vi "DimIndicators.VI-Tree.vi"   [LabVIEW 2014, in "DimIndicators.lvlib"]
doc: "DimIndicators provides some easy to use indicators and controls for GUIs.\n\nHistory: 21-FEB-2006, Dietrich Beck\n\nCopyright (C)\nGesellschaft für Schwerionenforschung, GSI\nPlanckstr. 1\n64291 Darmstadt\nGermany\n\nContact: D.Beck@gsi.de \n\nThis program is free software; you can redistribute it and/or modify it under the terms of the GNU General Public License as published by the Free Software Foundation; either version 2 of the license, or (at your option) any later version.\n\nThis program is distributed in the hope that it will be useful, but WITHOUT ANY WARRANTY; without even the implied warranty of MERCHANTABILITY or FITNESS FOR A PARTICULAR PURPOSE. See the GNU General License for more details (http://www.gnu.org).\n\nGesellschaft für Schwerionenforschung, GSI\nPlanckstr. 1, 64291 Darmstadt, Germany\nFor all questions and ideas contact D. Beck.\nLast update: 16-DEC-2005"
uses:
  DimIndicators.lvlib
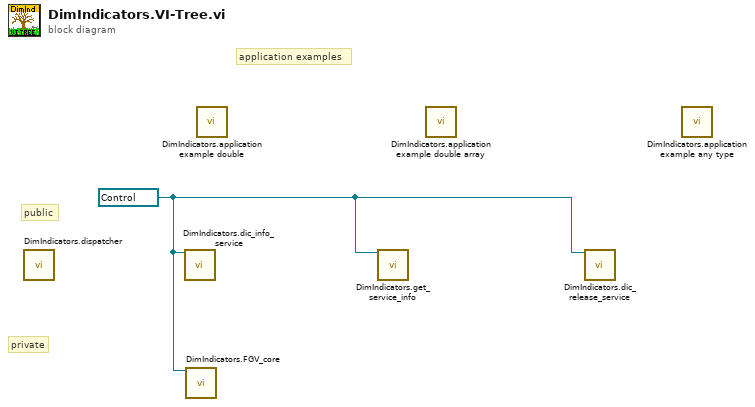
[diagram p0: block diagram]
diagram:
  w1 = refnum<vi> refnum ("controlRef")
  # "private"
  # "public"
  # "application examples"
  n1 = call "DimIndicators.dispatcher.vi"() -> ()  [unwired: 12 in]
  n2 = call "DimIndicators.dic_info_service.vi"("controlRef"=w1) -> ()  [unwired: 17 in, 2 out]
  n3 = call "DimIndicators.FGV_core.vi"("controlRef"=w1) -> ()  [unwired: 15 in, 4 out]
  n4 = call "DimIndicators.application example double.vi"() -> ()  [unwired: 1 in]
  n5 = call "DimIndicators.get_service_info.vi"("controlRef"=w1) -> ()  [unwired: 13 in, 6 out]
  n6 = call "DimIndicators.application example double array.vi"() -> ()  [unwired: 1 in]
  n7 = call "DimIndicators.dic_release_service.vi"("controlRef"=w1) -> ()  [unwired: 18 in, 1 out]
  n8 = call "DimIndicators.application example any type.vi"() -> ()  [unwired: 1 in]
